vi "ZCalibration V2.vi"(9 "xi":dbl[](array[numeric]) format="%_6g", 10 "Field of View":u16(ring) items=["130", "175", "260"], 11 "Objective":u16(ring)=1 items=["25X", "40X"]) -> (1 "Zmin value":dbl, 2 "Zmax value":dbl, 3 "yi":dbl[](array[numeric]) format="%_6g")   [LabVIEW 2020]
uses:
  <vilib>/gmath/NI_Gmath.lvlib
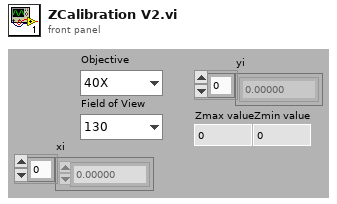
[diagram p1: front panel]
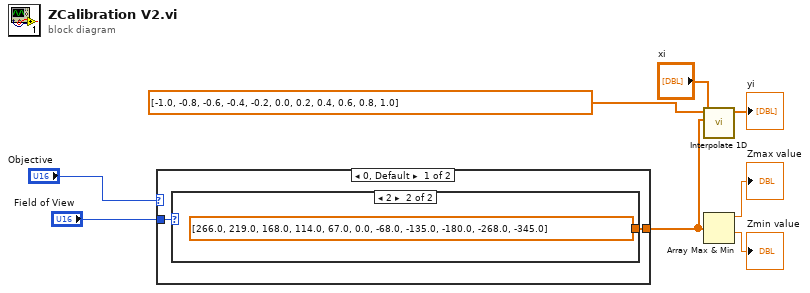
[diagram p0: block diagram]
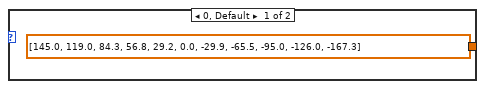
[diagram p2: hidden frame]
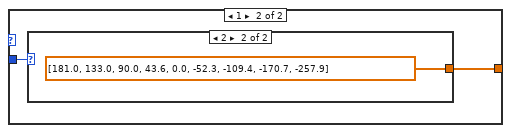
[diagram p3: hidden frame]
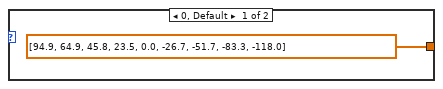
[diagram p4: hidden frame]
diagram:
  n1 = case shown="0, Default" "Objective" {
    tunnel: "Field of View" -> [w9 w14]
    tunnel: [w10 w13] -> w2
    frame 0, Default {
      n2 = case shown="2" w9 {
        tunnel: [dbl[] [145.0, 119.0, 84.3, 56.8, 29.2, 0.0, -29.9, -65.5, -95.0, -126.0, -167.3] dbl[] [266.0, 219.0, 168.0, 114.0, 67.0, 0.0, -68.0, -135.0, -180.0, -268.0, -345.0]] -> w10
        frame 0, Default {
        }
        frame 2 {
        }
      }
    }
    frame 1 {
      n3 = case shown="2" w14 {
        tunnel: [dbl[] [94.9, 64.9, 45.8, 23.5, 0.0, -26.7, -51.7, -83.3, -118.0] dbl[] [181.0, 133.0, 90.0, 43.6, 0.0, -52.3, -109.4, -170.7, -257.9]] -> w13
        frame 0, Default {
        }
        frame 2 {
        }
      }
    }
  }
  n4 = call <vilib>:"Interpolate 1D.vi"("xi"="xi", "X"=w2, "Y"=dbl[] [-1.0, -0.8, -0.6, -0.4, -0.2, 0.0, 0.2, 0.4, 0.6, 0.8, 1.0]) -> ("yi"=→"yi":dbl[])  [unwired: 6 in, 2 out]
  n5 = Array Max & Min(array=w2) -> (max value=→"Zmax value":dbl, min value=→"Zmin value":dbl)  [unwired: 2 out]
